vi "generateSignedUUIDs.vi"(6 "timeout (10000)":i32=10000, 8 "error in (no error)":errorcluster, 11 "Parameters":T2) -> (0 "error out":errorcluster, 3 "Response":T1, 4 "error data":string[](array[string]))   [LabVIEW 2014, in "Random JSON API.lvlib"]
uses:
  Random JSON API.lvlib
  Type Defs/generateUUIDsRequest.ctl
  Type Defs/generateSignedUUIDsResponse.ctl
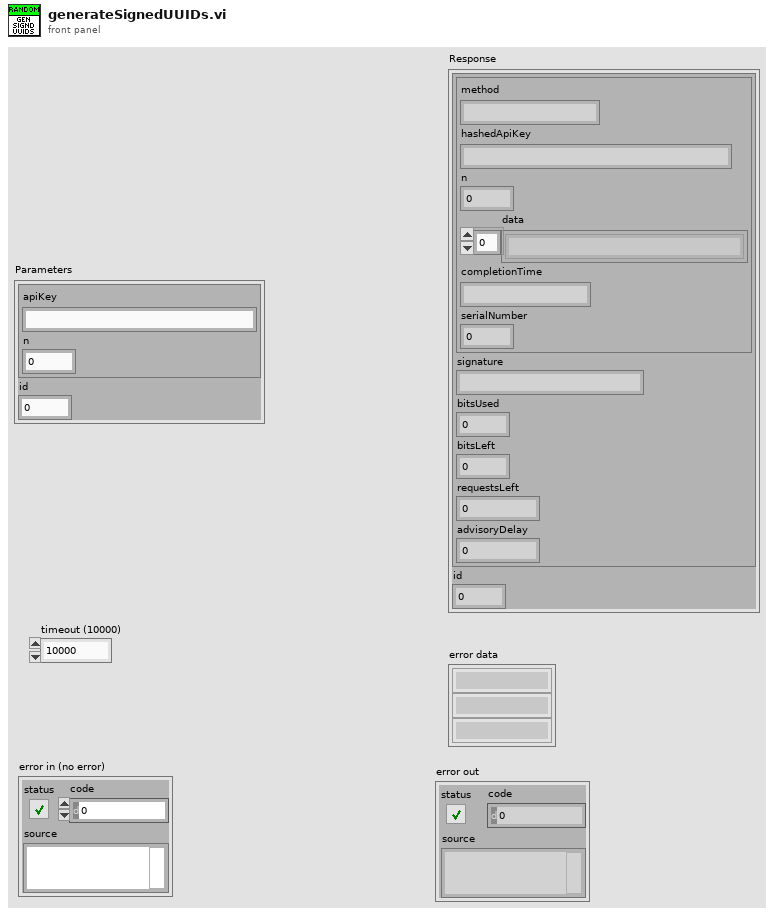
[diagram p1: front panel]
types:
  T1 = typedef "Random JSON API.lvlib/generateSignedUUIDsResponse.ctl" = cluster{"result":cluster{"random":cluster{"method":string, "hashedApiKey":string, "n":i32, "data":string[], "completionTime":string, "serialNumber":i32}, "signature":string, "bitsUsed":i32, "bitsLeft":i32, "requestsLeft":i32, "advisoryDelay":i32}, "id":dbl}
  T2 = typedef "Random JSON API.lvlib/generateUUIDsRequest.ctl" = cluster{"params":cluster{"apiKey":string, "n":i32}, "id":dbl}
  T3 = cluster{"jsonrpc":string, "method":string, "params":cluster{"apiKey":string, "n":i32}, "id":dbl}
  T4 = cluster{"result cluster":cluster{"completionTime":string, "bitsUsed":i32, "bitsLeft":i32, "requestsLeft":i32, "advisoryDelay":i32}, "method":string, "hashedApiKey":string, "n":i32, "serialNumber":i32, "signature":string}
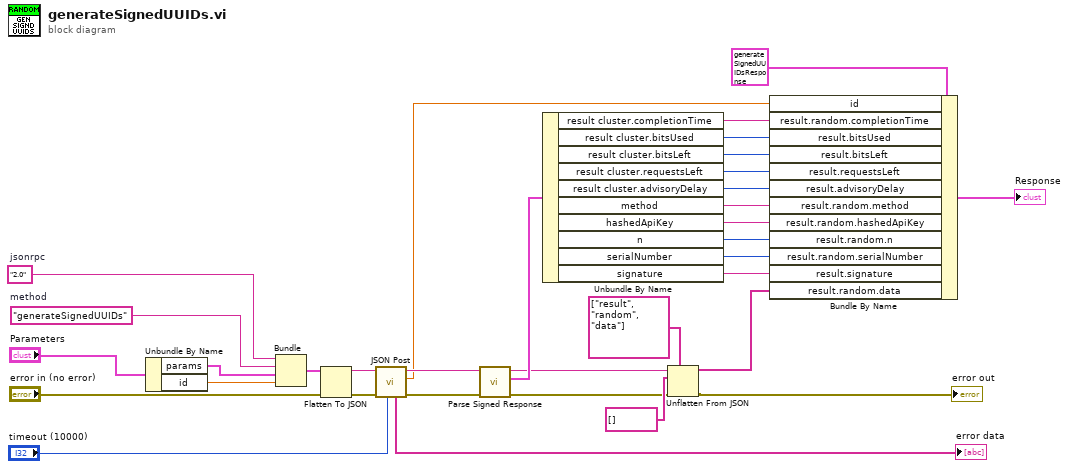
[diagram p0: block diagram]
diagram:
  w23 = "2.0"  # jsonrpc
  w22 = "generateSignedUUIDs"  # method
  n1 = Unbundle By Name("Parameters") -> ("params"=w21:cluster{"apiKey":string, "n":i32}, "id"=w20:dbl)
  n2 = Bundle("jsonrpc"=w23, "method"=w22, "params"=w21, "id"=w20) -> (w19:T3)  [unwired: 1 in]
  n3 = Flatten To JSON(anything=w19, error in (no error)="error in (no error)") -> (JSON string=w26:string, 11:w25:errorcluster)  [unwired: 1 in]
  n4 = call "JSON Post.vi"("timeout (10000)"="timeout (10000)", "error in (no error)"=w25, "Request JSON String"=w26) -> ("error out"=w32:errorcluster, "id"=w13:dbl, "Response JSON String"=w14:string, "error data"=→"error data":string[])  [unwired: 5 in]
  n5 = call "Parse Signed Response.vi"("error in (no error)"=w32, "body in"=w14) -> ("error out"=w10:errorcluster, "signed result cluster"=w15:T4, "body out"=w12:string)  [unwired: 7 in]
  n6 = Unbundle By Name(w15) -> ("result cluster.completionTime"=w31:string, "result cluster.bitsUsed"=w30:i32, "result cluster.bitsLeft"=w29:i32, "result cluster.requestsLeft"=w28:i32, "result cluster.advisoryDelay"=w27:i32, "method"=w5:string, "hashedApiKey"=w4:string, "n"=w3:i32, "serialNumber"=w2:i32, "signature"=w1:string)
  n7 = Unflatten From JSON(path=string[] ["result", "random", "data"], JSON string=w12, type and defaults=string[] [], error in (no error)=w10) -> (value=w6:string[], error out=→"error out":errorcluster)  [unwired: 3 in]
  n8 = Bundle By Name(cluster=T1 {"result"={"random"={"method"="", "hashedApiKey"="", "n"=0, "data"=[], "completionTime"="", "serialNumber"=0}, "signature"="", "bitsUsed"=0, "bitsLeft"=0, "requestsLeft"=0, "advisoryDelay"=0}, "id"=0.0} ("Response"), "id"=w13, "result.random.completionTime"=w31, "result.bitsUsed"=w30, "result.bitsLeft"=w29, "result.requestsLeft"=w28, "result.advisoryDelay"=w27, "result.random.method"=w5, "result.random.hashedApiKey"=w4, "result.random.n"=w3, "result.random.serialNumber"=w2, "result.signature"=w1, "result.random.data"=w6) -> (→"Response":T1)
